vi "configure offset.vi"(7 "offset_val2":u32, 8 "error in (no error)":errorcluster, 9 "offset_val1":u32, 10 "Board":u16, 11 "identifier":string) -> (0 "error out":errorcluster, 3 "function return":u32)   [LabVIEW 2015, in "XGL_DPP.lvlib"]
doc: "EXTERN DECLSPEC uint32_t CALL_CONV configure_offset(const char * identifier, uint16_t Board, const configuration_offset cfg_offset);"
uses:
  XGL_DPP.lvlib
  XGL_DPP.dll
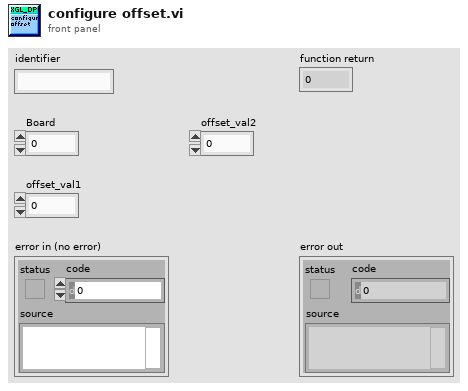
[diagram p1: front panel]
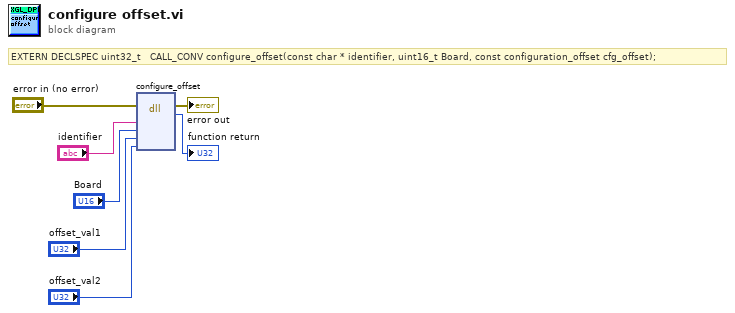
[diagram p0: block diagram]
diagram:
  # "EXTERN DECLSPEC uint32_t   CALL_CONV configure_offset(const char * identifier, uint16_t Board, const configuration_offset cfg_offset);"
  n1 = dll-call lib="D:/Users/XRF/Desktop/Scanning Software_Demokritos_2015_v7/libs/Vis_2/XGL_DPP.*" fn="configure_offset"(error in="error in (no error)", "identifier"="identifier", "Board"="Board", "offset_val1"="offset_val1", "offset_val2"="offset_val2") -> (error out=→"error out":errorcluster, →"function return":u32)  [unwired: 6 in, 1 out]
